vi "XPS positions FGV.vi"(8 "error in":errorcluster, 10 "Function":T2, 11 "Acq Data in":T1) -> (0 "error out":errorcluster, 3 "Acq Data out":T1)   [LabVIEW 2020]
uses:
  XPS Acquire FGV.ctl
  stop FGV control.ctl
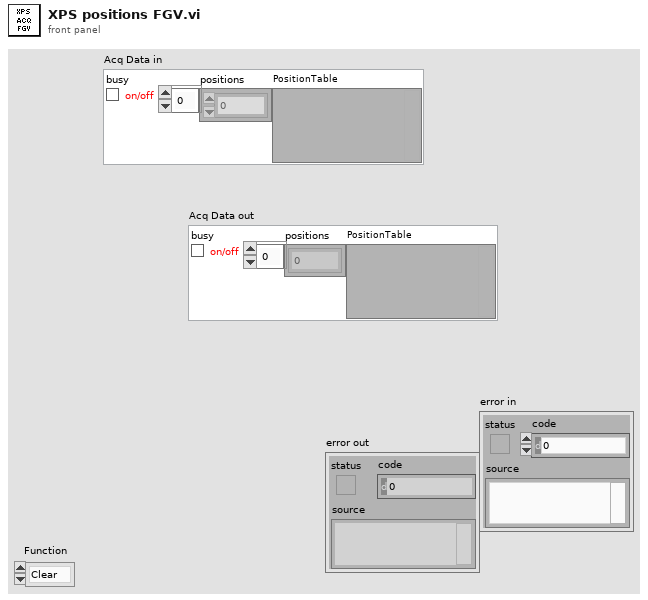
[diagram p1: front panel]
types:
  T1 = typedef "XPS Acquire FGV.ctl" = cluster{"busy":bool, "positions":dbl[], "PositionTable":variant}
  T2 = typedef "stop FGV control.ctl" = enum16{"Clear", "Write", "Read"}
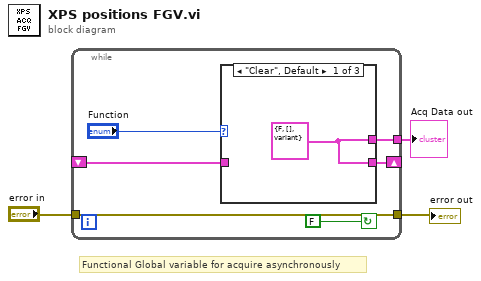
[diagram p0: block diagram]
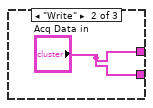
[diagram p2: hidden frame]
diagram:
  # "Functional Global variable for acquire asynchronously"
  n1 = while {
    shift-left: _ -> [w8]
    shift-right: [w9] -> _
    tunnel: [w5] -> w1
    tunnel: "error in" -> [w4]
    tunnel: [w4] -> w2
    stop <- FALSE continue-if-true
    n2 = case shown="\"Clear\", Default" "Function" {
      tunnel: [w10 "Acq Data in" w12] -> w9
      tunnel: w8 -> [_ _ w12]
      tunnel: [w10 "Acq Data in" w12] -> w5
      frame "Clear", Default {
        w10 = T1 {"busy"=FALSE, "positions"=[], "PositionTable"=variant} ("ESP301 Acq Data 2")
      }
      frame "Write" {
      }
      frame "Read" {
      }
    }
  }
  "error out" <- w2
  "Acq Data out" <- w1
